vi "iXonEMCCD_Cool_Off.vi"() -> ()   [LabVIEW 2025]
panel:
  out "Cool Off ?":bool
  out "Current Temperature":i32
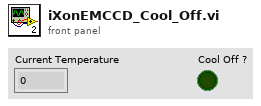
[diagram p1: front panel]
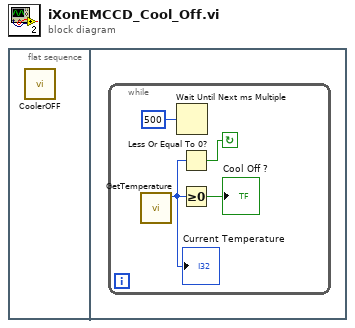
[diagram p0: block diagram]
diagram:
  n1 = flat-sequence {
    frame #0 {
      n2 = call "CoolerOFF.vi"() -> ()  [unwired: 2 in, 2 out]
    }
    frame #1 {
      n3 = while {
        stop <- w3 continue-if-true
        n4 = call "GetTemperature.vi"() -> ("temperature"=w1:i32)  [unwired: 4 in, 3 out]
        "Current Temperature" <- w1
        n5 = Wait Until Next ms Multiple(millisecond multiple=u32 500) -> ()  [unwired: 1 out]
        n6 = Less Or Equal To 0?(x=w1) -> (x <= 0?=w3:bool)
        n7 = Greater Or Equal To 0?(x=w1) -> (x >= 0?=→"Cool Off ?":bool)
      }
    }
  }
